vi "根据起点终点角度计算搜索线.vi"(6 "从内外外搜索":bool, 7 "画搜索线?":bool, 8 "角度":dbl, 9 "Fitted Circle":T2, 10 "内径外径":cluster{"内径":dbl, "外径":dbl}, 11 "Img in":T1) -> (0 "ROI 找边":T3 {"Contours"."Type" items=["No Selection", "Point", "Line", "Rectangle", "Oval", "Polygon", "Freehand Region", "Annulus", "Unused2", "Unused3", "Broken Line", "Freehand Line", "Rotated Rectangle"]}, 1 "找不到边界时默认点":cluster{dbl, dbl}, 3 "Img out":T1)   [LabVIEW 2014]
uses:
  <vilib>/vision/Image Controls.llb/IMAQ Image.ctl
panel:
  out "搜索线":cluster{cluster{dbl, dbl}, cluster{dbl, dbl}}
  out "从内往外搜索线":cluster{cluster{dbl, dbl}, cluster{dbl, dbl}}
  out "cos sin":cluster{dbl, dbl}
  out "从外往内搜索线":cluster{cluster{dbl, dbl}, cluster{dbl, dbl}}
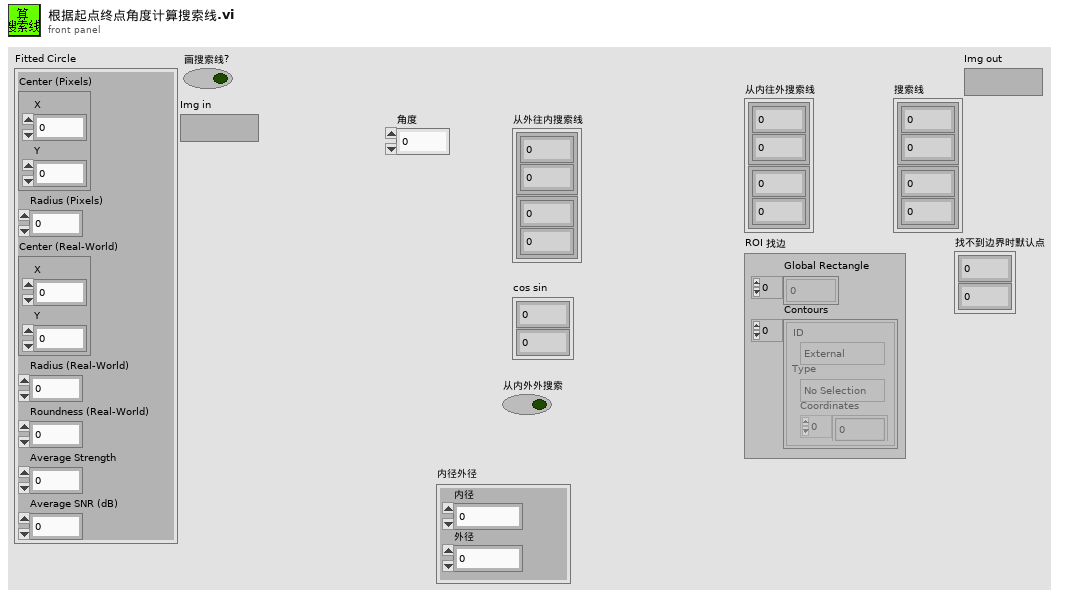
[diagram p1: front panel]
types:
  T1 = typedef "IMAQ Image.ctl" = refnum<image>
  T2 = cluster{"Center (Pixels)":cluster{"X":sgl, "Y":sgl}, "Radius (Pixels)":dbl, "Center (Real-World)":cluster{"X":sgl, "Y":sgl}, "Radius (Real-World)":dbl, "Roundness (Real-World)":dbl, "Average Strength":dbl, "Average SNR (dB)":dbl}
  T3 = typedef "ROI Descriptor" = cluster{"Global Rectangle":i32[], "Contours":cluster{"ID":enum32{"External", "Internal"}, "Type":u32, "Coordinates":i32[]}[]}
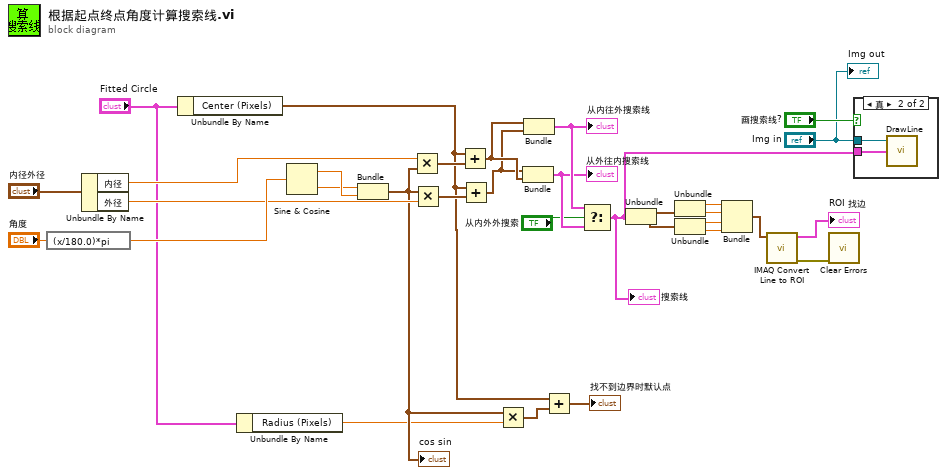
[diagram p0: block diagram]
diagram:
  n1 = expression code="(x/180.0)*pi" ("degrees to radians")("角度") -> (w27:dbl)
  n2 = Unbundle By Name("内径外径") -> ("内径"=w11:dbl, "外径"=w10:dbl)
  n3 = Unbundle By Name("Fitted Circle") -> ("Center (Pixels)"=w5:cluster{"X":sgl, "Y":sgl})
  n4 = Unbundle By Name("Fitted Circle") -> ("Radius (Pixels)"=w6:dbl)
  n5 = Sine & Cosine(0:w27) -> (1:w32:dbl, 2:w31:dbl)
  n6 = Bundle(w31, w32) -> (w8:cluster{dbl, dbl})  [unwired: 1 in]
  "cos sin" <- w8
  n7 = Multiply(x=w11, y=w8) -> (x*y=w29:cluster{dbl, dbl})
  n8 = Multiply(x=w8, y=w10) -> (x*y=w30:cluster{dbl, dbl})
  n9 = Add(x=w5, y=w29) -> (x+y=w26:cluster{dbl, dbl})
  n10 = Add(x=w5, y=w30) -> (x+y=w25:cluster{dbl, dbl})
  n11 = Multiply(x=w8, y=w6) -> (x*y=w9:cluster{dbl, dbl})
  n12 = Bundle(w25, w26) -> (w17:cluster{cluster{dbl, dbl}, cluster{dbl, dbl}})  [unwired: 1 in]
  "从外往内搜索线" <- w17
  n13 = Bundle(w26, w25) -> (w18:cluster{cluster{dbl, dbl}, cluster{dbl, dbl}})  [unwired: 1 in]
  "从内往外搜索线" <- w18
  n14 = Add(x=w5, y=w9) -> (x+y=→"找不到边界时默认点":cluster{dbl, dbl})
  n15 = Select(t=w18, s="从内外外搜索", f=w17) -> (s? t:f=w3:cluster{cluster{dbl, dbl}, cluster{dbl, dbl}})
  "搜索线" <- w3
  n16 = Unbundle(w3) -> (w24:cluster{dbl, dbl}, w23:cluster{dbl, dbl})
  n17 = Unbundle(w24) -> (w22:dbl, w21:dbl)
  n18 = Unbundle(w23) -> (w20:dbl, w19:dbl)
  n19 = Bundle(w22, w21, w20, w19) -> (w15:cluster{dbl, dbl, dbl, dbl})  [unwired: 1 in]
  n20 = call "IMAQ Convert Line to ROI"("Line"=w15) -> ("error out"=w14:errorcluster, "ROI Descriptor"=→"ROI 找边":T3)  [unwired: 8 in]
  n21 = call <vilib>:"Clear Errors.vi"("error in (no error)"=w14) -> ()  [unwired: 5 in, 2 out]
  n22 = case shown="真" "画搜索线?" {
    tunnel: "Img in" -> [_ w34]
    tunnel: w3 -> [_ w33]
    frame False {
    }
    frame True {
      n23 = call "DrawLine.vi"("Edge Points"=w33, "img in"=w34) -> ()  [unwired: 1 in, 1 out]
    }
  }
  "Img out" <- "Img in"
